vi "Transform.vi"(7 "Type X":T1(ring), 8 "error in (no error)":errorcluster caption="entrée d'erreur (pas d'erreur)", 9 "y":string[][](array[string]), 10 "X":string[][](array[string]), 11 "GaussianRandomProjection.lvclass":refnum<class "GaussianRandomProjection.lvclass">) -> (0 "error out":errorcluster caption="sortie d'erreur", 2 "Data":T2, 3 "GaussianRandomProjection.lvclass":refnum<class "GaussianRandomProjection.lvclass">)   [LabVIEW 2020, in "GaussianRandomProjection.lvclass"]
doc: "Project the data by using matrix product with the random matrix\n\nReturns : \n\n- X_new : numpy array or scipy sparse of shape [n_samples, n_components]\nProjected array."
uses:
  GaussianRandomProjection.lvclass
  GaussianRandomProjection.lvclass/GaussianRandomProjection.ctl
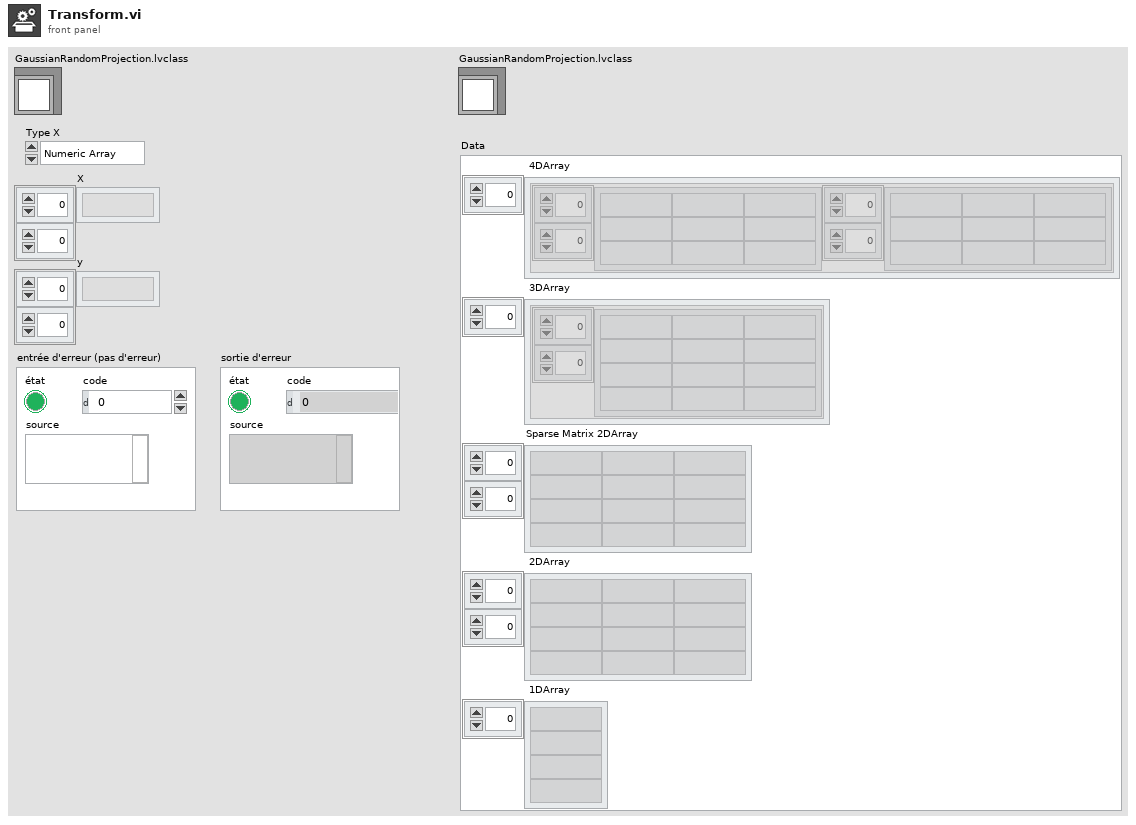
[diagram p1: front panel]
types:
  T1 = enum16{"Numeric Array", "String Array", "Sparse"}
  T2 = cluster{" 4DArray":cluster{"1":string[][], "2":string[][]}[], " 3DArray":cluster{"Tableau":string[][]}[], "Sparse Matrix 2DArray":string[][], " 2DArray":string[][], " 1DArray":string[]}
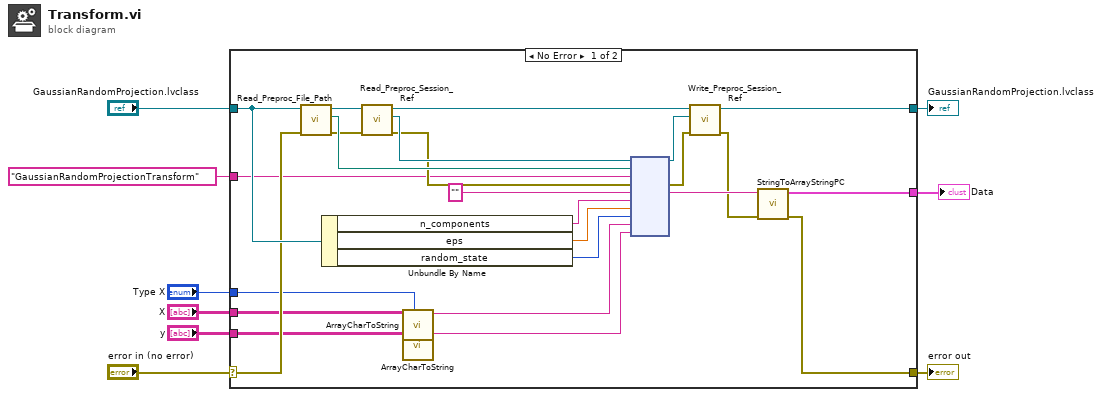
[diagram p0: block diagram]
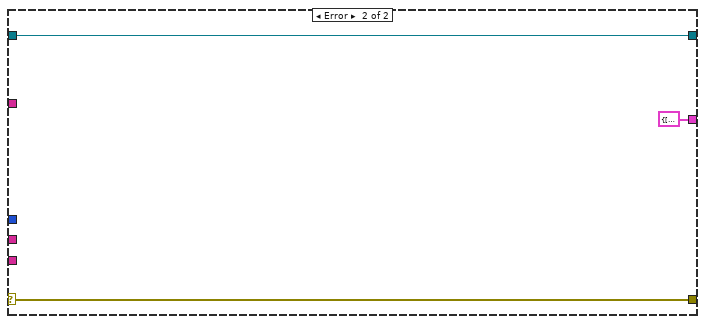
[diagram p2: hidden frame]
diagram:
  n1 = case shown="No Error" "error in (no error)" {
    selector: "error in (no error)" -> [w24 w35]
    tunnel: "GaussianRandomProjection.lvclass" -> [w25 w37]
    tunnel: "GaussianRandomProjectionTransform" ("Fonction") -> [w23 _]
    tunnel: [w17 T2 {" 4DArray"=[], " 3DArray"=[], "Sparse Matrix 2DArray"=[], " 2DArray"=[], " 1DArray"=[]} ("Data")] -> w4
    tunnel: "X" -> [w14 _]
    tunnel: "y" -> [w12 _]
    tunnel: [w19 w37] -> w3
    tunnel: [w15 w35] -> w2
    tunnel: "Type X" -> [w13 _]
    frame No Error {
      n2 = call-dynamic "Read_Preproc_File_Path.vi"("error in (no error)"=w24, "Python in"=w25) -> ("error out"=w29:errorcluster, "File_Path"=w32:path, "Python out"=w34:refnum<class "GaussianRandomProjection.lvclass">)  [unwired: 7 in]
      n3 = Unbundle By Name(w25) -> ("n_components"=w22:string, "eps"=w21:dbl, "random_state"=w20:i32)
      n4 = call-dynamic "Read_Preproc_Session_Ref.vi"("error in (no error)"=w29, "Python in"=w34) -> ("error out"=w30:errorcluster, "Session_ref"=w31:refnum<k35>, "Python out"=w33:refnum<class "GaussianRandomProjection.lvclass">)  [unwired: 7 in]
      n5 = call "ArrayCharToString.vi"("Type"=w13, "TAB"=w14) -> ("Instruction"=w10:string)  [unwired: 9 in]
      n6 = call "ArrayCharToString.vi"("TAB"=w12) -> ("Instruction"=w11:string)  [unwired: 10 in]
      n7 = node(w31, w32, w23, w30, "", w22, w21, w20, w10, w11) -> (w26:refnum<k35>, w28:errorcluster, w18:string)  [unwired: 5 in, 2 out]
      n8 = call-dynamic "Write_Preproc_Session_Ref.vi"("error in (no error)"=w28, "Session_ref"=w26, "Python in"=w33) -> ("error out"=w16:errorcluster, "Python out"=w19:refnum<class "GaussianRandomProjection.lvclass">)  [unwired: 7 in]
      n9 = call "StringToArrayStringPC.vi"("sortie d'erreur"=w16, "Return value"=w18) -> ("sortie d'erreur"=w15:errorcluster, "Data"=w17:T2)  [unwired: 8 in]
    }
    frame Error {
    }
  }
  "error out" <- w2
  "GaussianRandomProjection.lvclass" <- w3
  "Data" <- w4
